vi "SS2 Live_Check Valid Gate Definition.vi"(8 "Error In":errorcluster, 11 "SS2 DAQ Parameters in":T1 {"# Sets" min=1}) -> (0 "Error Out":errorcluster, 3 "SS2 DAQ Parameters out":T1 {"# Sets" min=1})   [LabVIEW 2019]
uses:
  SS2 DAQ Parameters 2.ctl
  SS2 Gate Definition.ctl
  SS2 Gate Configuration.ctl
  SS2 Live_Gate Configuration Action.ctl
  SS2 Live_Globals.vi
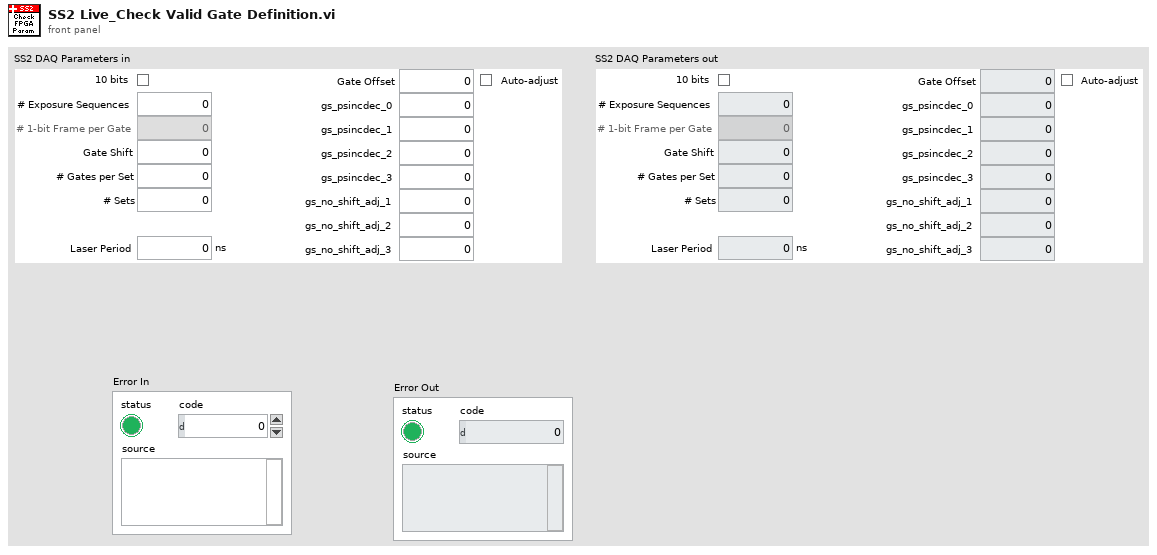
[diagram p1: front panel]
types:
  T1 = typedef "SS2 DAQ Parameters 2.ctl" = cluster{"10 bits":bool, "# Exposure Sequences":u32, "# 1-bit Frame per Gate":u32, "Gate Shift":u32, "# Gates per Set":u32, "# Sets":u32, "Laser Period":dbl[unit], "Gate Offset":u32, "Auto-adjust Gate Offset":bool, "Gate Definition":T2}
  T2 = typedef "SS2 Gate Definition.ctl" = cluster{"gs_psincdec_0":u32, "gs_psincdec_1":u32, "gs_psincdec_2":u32, "gs_psincdec_3":u32, "gs_no_shift_adj_1":u32, "gs_no_shift_adj_2":u32, "gs_no_shift_adj_3":u32}
  T3 = typedef "SS2 Live_Gate Configuration Action.ctl" = enum16{"Get Gate Configuration Name", "Get Configuration by Name", "Add Gate Configuration", "Delete Gate Configuration", "Rename Gate Configuration"}
  T4 = typedef "SS2 Gate Configuration.ctl" = cluster{"Gate Configuration":string, "Gate Offset":u32, "Gate Definition":T2}
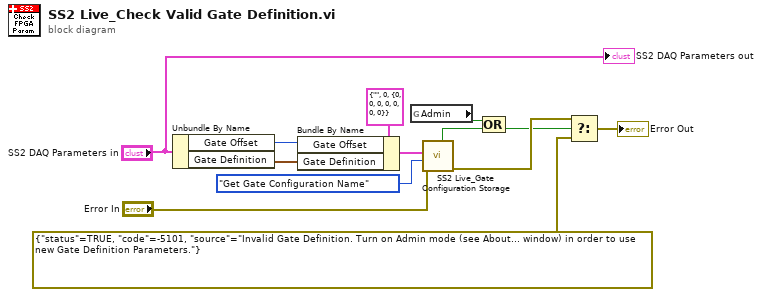
[diagram p0: block diagram]
diagram:
  n1 = Unbundle By Name("SS2 DAQ Parameters in") -> ("Gate Offset"=w11:u32, "Gate Definition"=w10:T2)
  n2 = Bundle By Name(cluster=T4 {"Gate Configuration"="", "Gate Offset"=0, "Gate Definition"={"gs_psincdec_0"=0, "gs_psincdec_1"=0, "gs_psincdec_2"=0, "gs_psincdec_3"=0, "gs_no_shift_adj_1"=0, "gs_no_shift_adj_2"=0, "gs_no_shift_adj_3"=0}} ("Gate Configuration Definition in"), "Gate Offset"=w11, "Gate Definition"=w10) -> (w12:T4)
  n3 = global read "SS2 Live_Globals.vi" "Admin"() -> (w2:bool)
  n4 = call "SS2 Live_Gate Configuration Storage.vi"("Error In"="Error In", "Action"=SS2_Live_Gate_Configuration_Action."Get Gate Configuration Name", "Gate Configuration Definition in"=w12) -> ("Error Out"=w5:errorcluster, "Gate Definition Found?"=w6:bool)  [unwired: 3 in, 4 out]
  n5 = Compound Arithmetic op=OR(w2, w6) -> (w3:bool)
  n6 = Select(t=w5, s=w3, f=errorcluster {"status"=TRUE, "code"=-5101, "source"="Invalid Gate Definition. Turn on Admin mode (see About... window) in order to use new Gate Definition Parameters."}) -> (s? t:f=→"Error Out":errorcluster)
  "SS2 DAQ Parameters out" <- "SS2 DAQ Parameters in"
